vi "Classify Error.vi"(10 "Error Code":i32) -> (2 "Error Classification":u32)   [LabVIEW 2014, in "Agilent ESA PSA Series.lvlib"]
doc: "This VI is used to check error code"
uses:
  Agilent ESA PSA Series.lvlib
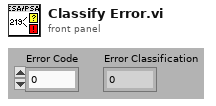
[diagram p1: front panel]
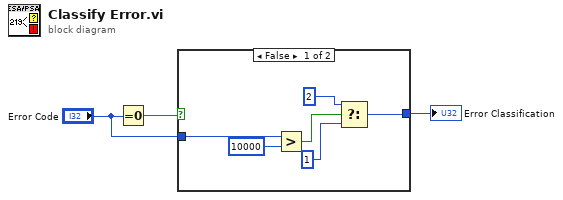
[diagram p0: block diagram]
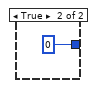
[diagram p2: hidden frame]
diagram:
  n1 = Equal To 0?(x="Error Code") -> (x = 0?=w3:bool)
  n2 = case shown="False" w3 {
    tunnel: [w4 0] -> w2
    tunnel: "Error Code" -> [w8 _]
    frame False {
      n3 = Greater?(x=w8, y=10000) -> (0:w9:bool)
      n4 = Select(t=2, s=w9, f=1) -> (s? t:f=w4:i32)
    }
    frame True {
    }
  }
  "Error Classification" <- w2
